vi "Get a Safe Token.vi"(10 "Index":i32, 11 "Constructor String Parser":T3) -> (2 "Failed Assert?":bool, 3 "Token":T1)   [LabVIEW 2020, in "Stream.lvlib" / "URLPattern.lvclass"]
uses:
  URLPattern.lvclass
  Token Type.ctl
  Token.ctl
  URL Pattern Init.ctl
  Parser State.ctl
  Constructor String Parser.ctl
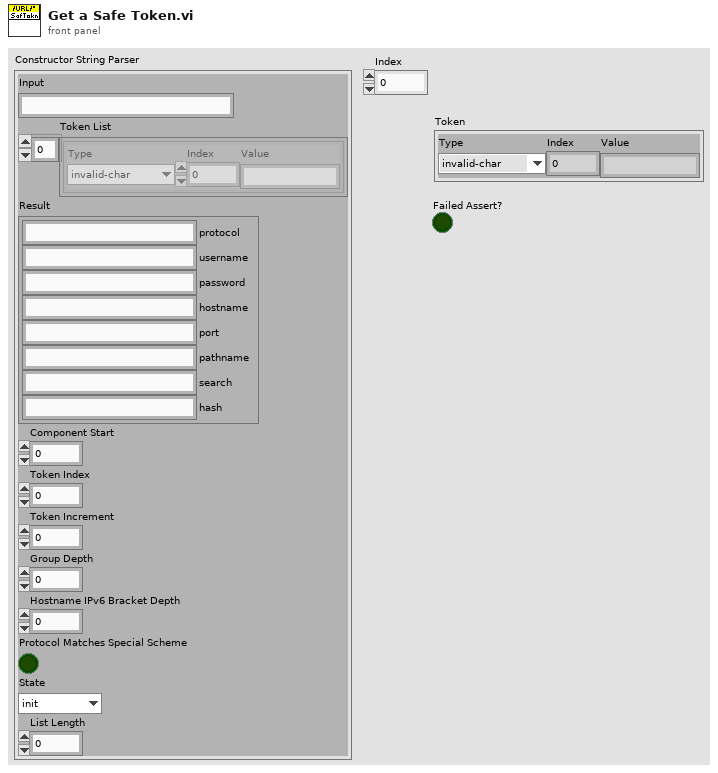
[diagram p1: front panel]
types:
  T1 = typedef "Stream.lvlib/URLPattern.lvclass/Token.ctl" = cluster{"Type":T2, "Index":i32, "Value":string}
  T2 = typedef "Stream.lvlib/URLPattern.lvclass/Token Type.ctl" = enum16{"invalid-char", "open", "close", "regexp", "name", "char", "escaped-char", "other-modifier", "asterisk", "end"}
  T3 = typedef "Stream.lvlib/URLPattern.lvclass/Constructor String Parser.ctl" = cluster{"Input":string, "Token List":T1[], "Result":T4, "Component Start":i32, "Token Index":i32, "Token Increment":i32, "Group Depth":i32, "Hostname IPv6 Bracket Depth":i32, "Protocol Matches Special Scheme":bool, "State":T5, "List Length":i32}
  T4 = typedef "Stream.lvlib/URLPattern.lvclass/URL Pattern Init.ctl" = cluster{"protocol":string, "username":string, "password":string, "hostname":string, "port":string, "pathname":string, "search":string, "hash":string}
  T5 = typedef "Stream.lvlib/URLPattern.lvclass/Parser State.ctl" = enum16{"init", "protocol", "authority", "username", "password", "hostname", "port", "pathname", "search", "hash", "done"}
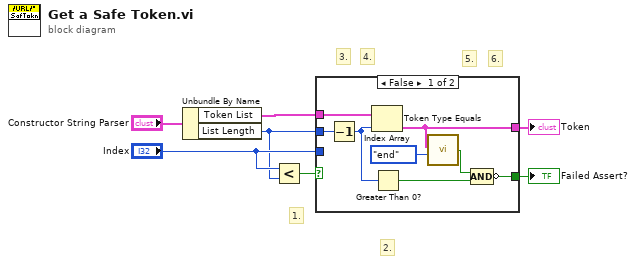
[diagram p0: block diagram]
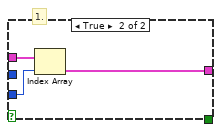
[diagram p2: hidden frame]
diagram:
  # "6."
  # "5."
  # "4."
  # "3."
  # "2."
  # "1."
  n1 = Unbundle By Name("Constructor String Parser") -> ("Token List"=w5:T1[], "List Length"=w2:i32)
  n2 = Less?(x="Index", y=w2) -> (x < y?=w6:bool)
  n3 = case shown="False" w6 {
    tunnel: w5 -> [w14 w18]
    tunnel: "Index" -> [_ w17]
    tunnel: [w8 w16] -> w3
    tunnel: w2 -> [w15 _]
    tunnel: [w11 _] -> w1
    frame False {
      n4 = Decrement(x=w15) -> (x-1=w13:i32)
      n5 = Index Array(array=w14, index=w13) -> (element=w8:T1)
      n6 = Greater Than 0?(x=w13) -> (x > 0?=w10:bool)
      n7 = call "Token Type Equals.vi"("Type"=Token_Type."end", "Token"=w8) -> ("Type Equals?"=w9:bool)  [unwired: 2 in]
      n8 = Compound Arithmetic op=AND(w9, w10) -> (invert w11:bool)
    }
    frame True {
      # "1."
      n9 = Index Array(array=w18, index=w17) -> (element=w16:T1)
    }
  }
  "Token" <- w3
  "Failed Assert?" <- w1
